vi "USB_VID.vi"(8 "error in (no error)":errorcluster, 10 "Parameters":string, 11 "reference in":refnum<class "Test_Flux_Capacitor.lvclass">) -> (0 "error out":errorcluster, 2 "Result":string, 3 "reference out":refnum<class "Test_Flux_Capacitor.lvclass">)   [LabVIEW 2022 SP3, in "Test_Flux_Capacitor.lvlib" / "Test_Flux_Capacitor.lvclass"]
uses:
  Test_Flux_Capacitor.lvclass
  <vilib>/JDP Science/JSONtext/JSONtext.lvlib
panel:
  in  "Parameter_Type":cluster{"default":string}
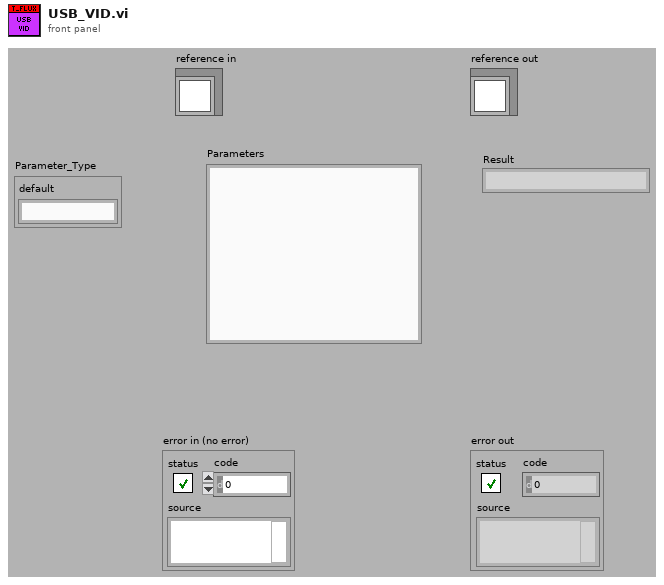
[diagram p1: front panel]
types:
  T1 = typedef "Test_Flux_Capacitor.lvlib/Test_Flux_Capacitor.lvclass/ObjectAttributes.ctl" = cluster{"Config":T2, "DMM":refnum<class "DMM_Keysight_34980A.lvclass">, "LCR":refnum<class "LCR_BK891.lvclass">, "PSU":refnum<class "PSU_Base.lvclass">, "Switch_Manager":refnum<class "SwitchBase.lvclass">, "FRAM":string, "Flux_Capacitor":refnum<class "Flux_Capacitor.lvclass">, "Frequency_Counter":refnum<class "Frequency_Counter_Base.lvclass">, "JTAG":refnum<class "JTAG_Base.lvclass">}
  T2 = typedef "Test_Flux_Capacitor.lvlib/Test_Flux_Capacitor.lvclass/Config.ctl" = cluster{"default":string}
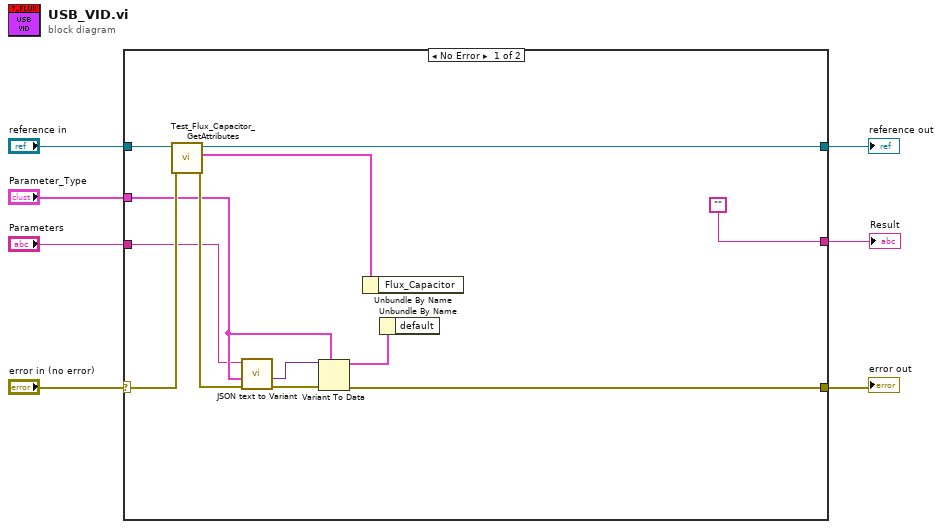
[diagram p0: block diagram]
diagram:
  n1 = case shown="No Error" "error in (no error)" {
    selector: "error in (no error)" -> [w19 w21]
    tunnel: [w9 w21] -> w6
    tunnel: [w15 w20] -> w4
    tunnel: "reference in" -> [w18 w20]
    tunnel: "Parameters" -> [w11 _]
    tunnel: "Parameter_Type" -> [w12 _]
    tunnel: ["" _] -> w1
    frame No Error {
      n2 = call "Test_Flux_Capacitor_GetAttributes.vi"("error in (no error)"=w19, "reference in"=w18) -> ("error out"=w14:errorcluster, "Data"=w17:T1, "reference out"=w15:refnum<class "Test_Flux_Capacitor.lvclass">)  [unwired: 6 in, 1 out]
      n3 = call <vilib>:"JSON text to Variant.vi"("error in (no error)"=w14, "Data Type"=w12, "JSON"=w11) -> ("error out"=w13:errorcluster, "Variant out"=w10:variant)  [unwired: 7 in]
      n4 = Variant To Data(error in=w13, type=w12, Variant=w10) -> (data=w16:cluster{"default":string}, error out=w9:errorcluster)
      n5 = Unbundle By Name(w17) -> ()  [unwired: 1 out]
      n6 = Unbundle By Name(w16) -> ()  [unwired: 1 out]
    }
    frame Error {
    }
  }
  "Result" <- w1
  "error out" <- w6
  "reference out" <- w4
